vi "Cleanup.vi"(8 "error in (no error)":errorcluster, 11 "DeviceDetailPanel in":refnum<class "DeviceDetailPanel.lvclass">) -> (0 "error out":errorcluster)   [LabVIEW 2020, in "PicoG-App.lvlib" / "DeviceDetailPanel.lvclass"]
uses:
  DeviceDetailPanel.lvclass
  <vilib>/IlluminatedG/IG OOPanel/OOPanel/Panel/Panel.lvclass
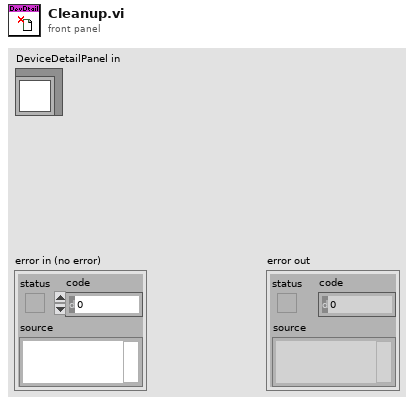
[diagram p1: front panel]
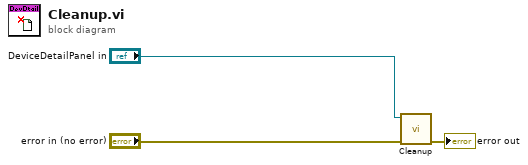
[diagram p0: block diagram]
diagram:
  n1 = call-parent "Cleanup.vi"("error in (no error)"="error in (no error)", "Panel in"="DeviceDetailPanel in") -> ("error out"=→"error out":errorcluster)  [unwired: 9 in]
